vi "getCurrentMode.vi"(8 "error":errorcluster, 11 "connection ID":refnum<k5>) -> (0 "error out":errorcluster, 2 "mode":string, 3 "connection ID out":refnum<k5>)   [LabVIEW 2016, in "sen_api.lvlib"]
doc: "Reads out the current device system state."
uses:
  sen_api.lvlib
panel:
  out "jsonRespIn":string
  out "JSON-response":string="{\"jsonrpc\":\"2.0\",\"method\":\"\",\"params\":[5,1.245,true,\"name\"],\"id\":\"1\"}"
  out "JSON request":string
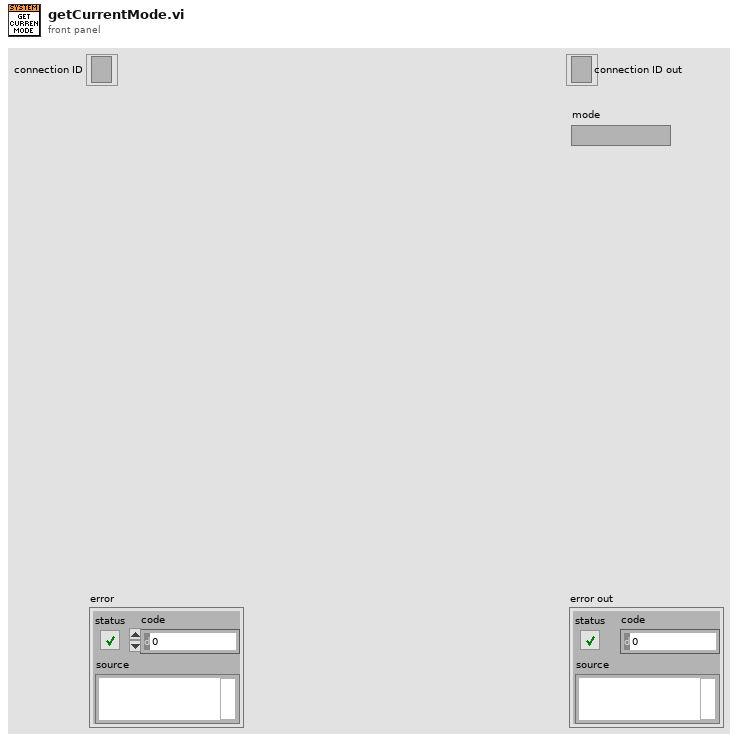
[diagram p1: front panel]
types:
  T1 = cluster{"jsonrpc":string, "method":string, "params":string[], "id":string, "api":i32, "pid":string}
  T2 = enum16{"Standard", "Buffered", "CRLF", "Immediate"}
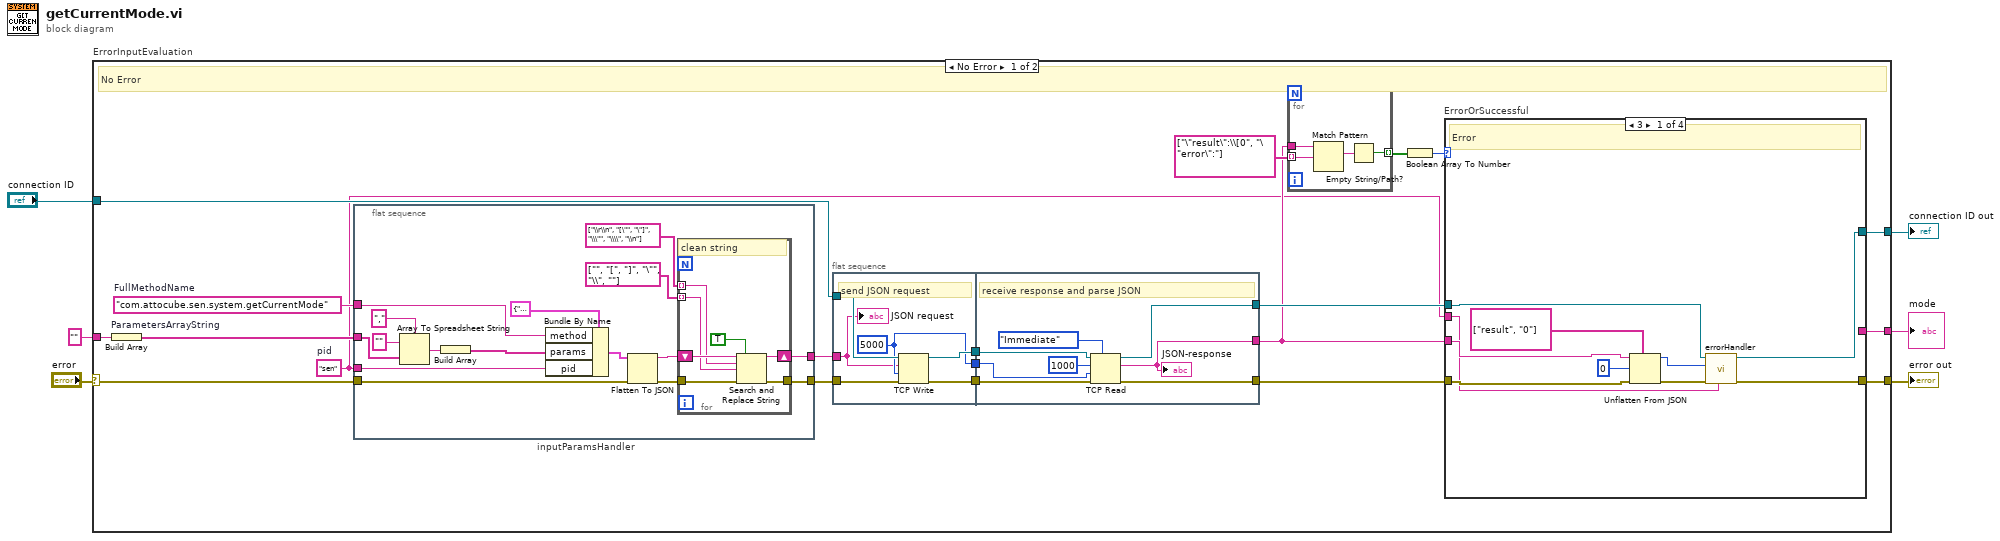
[diagram p0: block diagram]
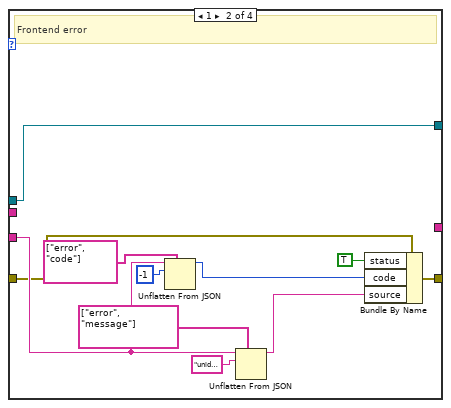
[diagram p2: hidden frame]
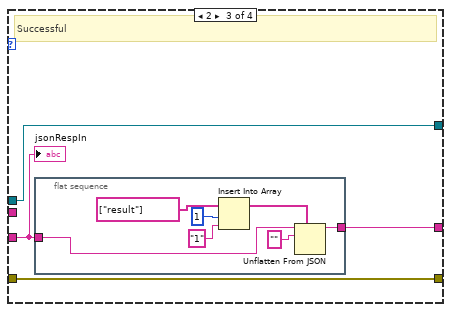
[diagram p3: hidden frame]
diagram:
  n1 = case "ErrorInputEvaluation" shown="No Error" "error" {
    selector: "error" -> [w13 w102]
    tunnel: "connection ID" -> [w23 w103]
    tunnel: [w15 w102] -> w5
    tunnel: [w16 w103] -> w4
    tunnel: "" -> [w8 _]
    tunnel: [w7 _] -> w1
    frame No Error {
      w9 = "sen"  # pid
      w14 = "com.attocube.sen.system.getCurrentMode"  # FullMethodName
      # "No Error"
      n2 = Build Array "ParametersArrayString"(w8) -> (w12:string[])
      n3 = flat-sequence "inputParamsHandler" {
        tunnel: [w30] -> w11
        tunnel: w12 -> [w37]
        tunnel: w13 -> [w35]
        tunnel: [w32] -> w10
        tunnel: w14 -> [w38]
        tunnel: w9 -> [w27]
        frame #0 {
          n4 = Array To Spreadsheet String(delimiter (Tab)=",", array=w37, 3:"" ("format string")) -> (spreadsheet string=w40:string)
          n5 = Build Array "Build Array"(w40) -> (w36:string[])
          n6 = Bundle By Name(cluster=T1 {"jsonrpc"="2.0", "method"="com.attocube.amc.res.setRESReadOutFreq", "params"=[], "id"="1", "api"=2, "pid"=""}, "method"=w38, "params"=w36, "pid"=w27) -> (w39:T1)
          n7 = Flatten To JSON(anything=w39, error in (no error)=w35) -> (JSON string=w31:string, 11:w33:errorcluster)  [unwired: 1 in]
          n8 = for {
            tunnel: string[] ["\\r\\n", "[\"", "\"]", "\\\"", "\\\\", "\\n"] ("search string") -> [w46] mode=indexing
            tunnel: string[] ["", "[", "]", "\"", "\\", ""] ("replace string (\"\")") -> [w45] mode=indexing
            shift-right: [w48] -> w30
            shift-left: w31 -> [w47]
            tunnel: w33 -> [w44]
            tunnel: [w43] -> w32
            # "clean string"
            n9 = Search and Replace String(replace all?=TRUE ("replace all? (F)"), input string=w47, search string=w46, replace string=w45, error in=w44) -> (result string=w48:string, error out=w43:errorcluster)  [unwired: 3 in, 2 out]
          }
        }
      }
      n10 = flat-sequence {
        tunnel: w23 -> [w93]
        tunnel: [w91] -> w26
        tunnel: [w92] -> w25
        tunnel: w10 -> [w88]
        tunnel: [w90] -> w24
        tunnel: w11 -> [w89]
        tunnel: [w97] -> w19
        tunnel: w26 -> [w99]
        tunnel: w25 -> [w98]
        tunnel: [w95] -> w18
        tunnel: w24 -> [w96]
        tunnel: [w94] -> w17
        frame #0 {
          w90 = 5000 ("timeout ms (25000)")
          # "send JSON request"
          n11 = TCP Write(connection ID=w93, data in=w89, error in (no error)=w88, 9:w90) -> (connection ID out=w91:refnum<k5>, error out=w92:errorcluster)  [unwired: 1 out]
          "JSON request" <- w89
        }
        frame #1 {
          # "receive response and parse JSON"
          n12 = TCP Read(connection ID=w99, bytes to read=1000, error in (no error)=w98, 7:T2."Immediate" ("mode (standard)"), 9:w96) -> (connection ID out=w97:refnum<k5>, data out=w94:string, error out=w95:errorcluster)
          "JSON-response" <- w94
        }
      }
      n13 = for {
        tunnel: string[] ["\"result\":\\[0", "\"error\":"] ("path") -> [w52] mode=indexing
        tunnel: [w50] -> w21 mode=indexing
        tunnel: w17 -> [w53]
        n14 = Match Pattern(string=w53, regular expression=w52) -> (match substring=w51:string)  [unwired: 1 in, 3 out]
        n15 = Empty String/Path?(string/path=w51) -> (empty?=w50:bool)
      }
      n16 = Boolean Array To Number(Boolean array=w21) -> (number=w20:u32)
      n17 = case "ErrorOrSuccessful" shown="3" w20 {
        tunnel: w17 -> [w57 w66 w76 _]
        tunnel: w19 -> [w61 w64 w78 w87]
        tunnel: [w59 w64 w78 w87] -> w16
        tunnel: [w60 w67 w77 w86] -> w15
        tunnel: w18 -> [w63 w65 w77 w86]
        tunnel: w9 -> [w54 _ _ _]
        tunnel: [_ _ w75 _] -> w7
        frame 3 {
          # "Error"
          n18 = Unflatten From JSON(path=string[] ["result", "0"], JSON string=w57, type and defaults=0, error in (no error)=w63) -> (value=w55:i32, error out=w62:errorcluster)  [unwired: 3 in]
          n19 = call "errorHandler.vi"("pid"=w54, "error in"=w62, "errNbr"=w55, "connection ID"=w61) -> ("error out 2"=w60:errorcluster, "connection ID out"=w59:refnum<k5>)  [unwired: 6 in]
        }
        frame 1 {
          # "Frontend error"
          n20 = Unflatten From JSON(path=string[] ["error", "code"], JSON string=w66, type and defaults=-1) -> (value=w73:i32)  [unwired: 4 in, 1 out]
          n21 = Unflatten From JSON(path=string[] ["error", "message"], JSON string=w66, type and defaults="unidentified error") -> (value=w74:string)  [unwired: 4 in, 1 out]
          n22 = Bundle By Name(cluster=w65, "status"=TRUE, "code"=w73, "source"=w74) -> (w67:errorcluster)
        }
        frame 2 {
          # "Successful"
          n23 = flat-sequence "out_string" {
            tunnel: w76 -> [w85]
            tunnel: [w79] -> w75
            frame #0 {
              n24 = Insert Into Array(array=string[] ["result"] ("path"), index=1, new element="1" ("idx")) -> (w82:string[])
              n25 = Unflatten From JSON(path=w82, JSON string=w85, type and defaults="") -> (value=w79:string)  [unwired: 4 in, 1 out]
            }
          }
          "jsonRespIn" <- w76
        }
        frame Default {
          # "NoResponse"
        }
      }
    }
    frame Error {
      # "Error"
    }
  }
  "error out" <- w5
  "connection ID out" <- w4
  "mode" <- w1
